vi "保存原始记录.vi"(8 "错误输入（无错误）":errorcluster, 11 "NI_report输入":refnum<class "NI_report.lvclass">) -> (0 "错误输出":errorcluster)   [LabVIEW 2015]
uses:
  <vilib>/Utility/NIReport.llb/NI_report.lvclass
  <vilib>/addons/_office/excel.llb/Excel Get Data (str).vi
  Global.vi
  <vilib>/addons/_office/NI_ReportGenerationToolkit.lvlib
  <vilib>/Utility/NIReport.llb/Excel/NI_Excel.lvclass
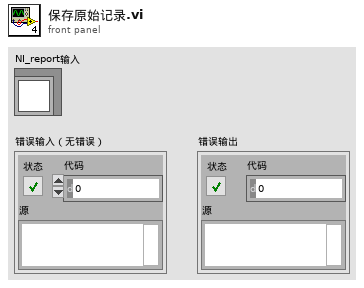
[diagram p1: front panel]
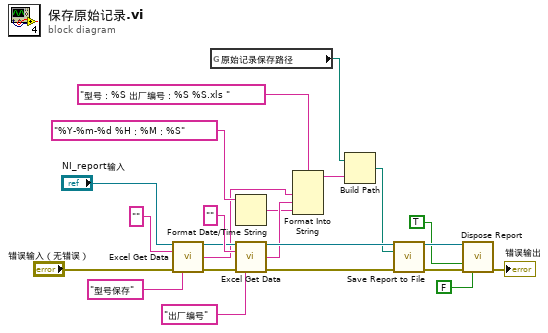
[diagram p0: block diagram]
diagram:
  n1 = call-poly <vilib>:"Excel Get Data.vi"("report in"="NI_report输入", "data type"="", "error in (no error)"="错误输入（无错误）", "name (\"\")"="型号保存" ("name (\"\")")) -> ("report out"=w20:refnum<class "NI_report.lvclass">, "data"=w10:string, "error out"=w21:errorcluster)  [unwired: 9 in]
  n2 = global read "Global.vi" "原始记录保存路径"() -> (w7:path)
  n3 = Format Date/Time String(time format string (%c)="%Y-%m-%d %H：%M：%S" ("时间格式字符串(%c)")) -> (date/time string=w8:string)  [unwired: 2 in]
  n4 = call-poly <vilib>:"Excel Get Data.vi"("report in"=w20, "data type"="", "error in (no error)"=w21, "name (\"\")"="出厂编号" ("name (\"\")")) -> ("report out"=w14:refnum<class "NI_report.lvclass">, "data"=w9:string, "error out"=w13:errorcluster)  [unwired: 9 in]
  n5 = Format Into String(format string="型号：%S 出厂编号：%S %S.xls " ("格式字符串"), w10, w9, w8) -> (resulting string=w6:string)  [unwired: 2 in, 1 out]
  n6 = Build Path(base path=w7, name or relative path=w6) -> (appended path=w5:path)
  n7 = call-dynamic "Save Report to File.vi"("report in"=w14, "report file path"=w5, "error in (no error)"=w13) -> ("report out"=w4:refnum<class "NI_report.lvclass">, "error out"=w3:errorcluster)  [unwired: 11 in]
  n8 = call-dynamic "Dispose Report.vi"("report in"=w4, "save changes? (F)"=TRUE, "error in (no error)"=w3, "close report? (T)"=FALSE ("save changes? (F)")) -> ("error out"=→"错误输出":errorcluster)  [unwired: 11 in]
